vi "isProcessAllowedRun.vi"(8 "error in (no error)":errorcluster, 11 "SMO in":refnum<class "SMO.lvclass">) -> (0 "error out":errorcluster, 2 "Run Allowed":bool, 3 "SMO out":refnum<class "SMO.lvclass">)   [LabVIEW 2013, in "SMO.lvclass"]
uses:
  SMO.lvclass
  SMO.lvclass/SMO.ctl
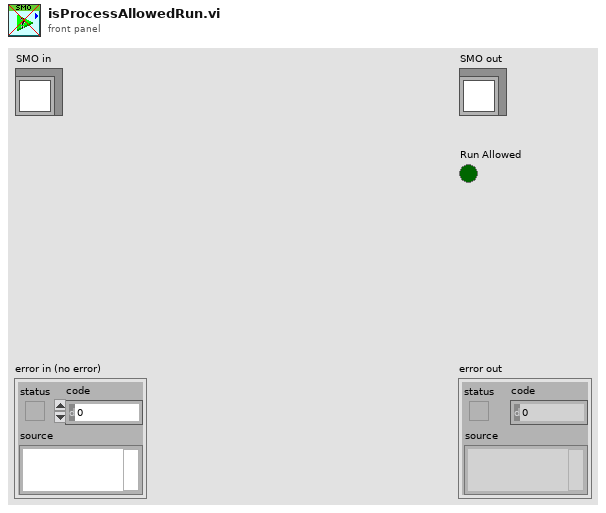
[diagram p1: front panel]
types:
  T1 = typedef "SMO.lvclass/PrivateData--Ref.ctl" = refnum<data-value>
  T2 = typedef "SMO.lvclass/PrivateData--Cluster.ctl" = cluster{"Parent Call":T3, "Registered Processes":T4[], "Sync Notifier":refnum<notifier>, "Process Error Notifier":refnum<notifier>, "Protected Events":T5, "Public Events":T6, "SMO State":T7, "[Dependencies]":T8[], "[Attributes]":refnum<class "Attribute.lvclass">[], "Launcher Close":refnum<notifier>}
  T3 = typedef "SMO.lvclass/Parent Call--Enum.ctl" = enum16{"Allows parent to run", "Does not request parent to run"}
  T4 = typedef "SMO.lvclass/RegisteredProcessData--Cluster.ctl" = cluster{"Name":string, "Static VI Ref":refnum<vi>, "Running":bool, "NotifierRef":u32}
  T5 = typedef "SMO.lvclass/Protected Events.ctl" = cluster{"StopProcesses":refnum<user-event>, "AbortProcesses":refnum<user-event>, "Config Changed":refnum<user-event>}
  T6 = typedef "SMO.lvclass/Public Events.ctl" = cluster{"Error":refnum<user-event>, "State":refnum<user-event>}
  T7 = typedef "SMO.lvclass/SMOState --Enum.ctl" = enum16{"unknown", "Created", "Started", "Stopped"}
  T8 = typedef "SMO.lvclass/SMO Dependency--Cluster.ctl" = cluster{"Dependency":refnum<class "SMO.lvclass">, "Level":string}
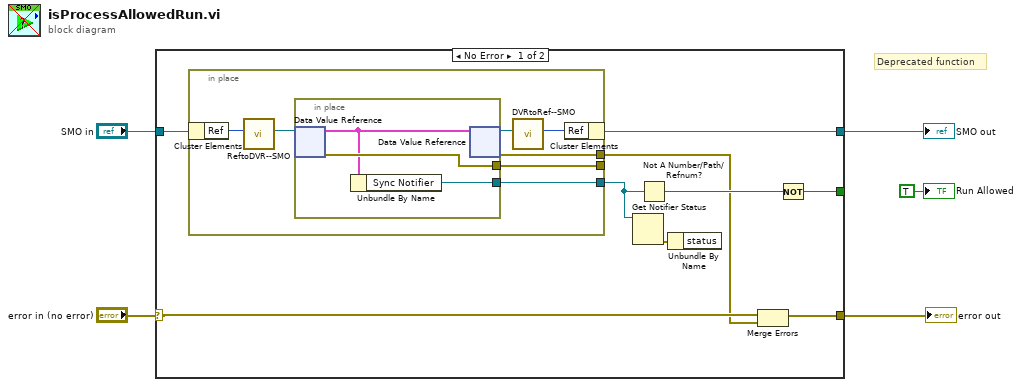
[diagram p0: block diagram]
diagram:
  # "Deprecated function"
  n1 = case shown="No Error" "error in (no error)" {
    selector: "error in (no error)" -> [w10 w26]
    tunnel: [w8 w26] -> w3
    tunnel: [w13 w25] -> w2
    tunnel: "SMO in" -> [w14 w25]
    tunnel: [w11 _] -> _
    frame No Error {
      n2 = in-place {
        in-place-border: [w21] -> w9
        in-place-border: [w20] -> _
        in-place-border: [w15] -> w7
        n3 = in-place-cluster #1(w14) -> ("Ref"=w19:u32)
        n4 = call "ReftoDVR--SMO.vi"("Ref"=w19) -> ("Ref"=w18:T1)  [unwired: 10 in]
        n5 = in-place {
          in-place-border: [w24] -> w20
          in-place-border: [w22] -> w15
          n6 = in-place-dvr #2(w18) -> (w23:T2, w24:errorcluster)
          n7 = Unbundle By Name(w23) -> ("Sync Notifier"=w22:refnum<notifier>)
          n8 = in-place-dvr #2(w23) -> (w17:T1, w21:errorcluster)
        }
        n9 = call "DVRtoRef--SMO.vi"("Ref"=w17) -> ("Ref"=w16:u32)  [unwired: 10 in]
        n10 = in-place-cluster #1("Ref"=w16) -> (w13:refnum<class "SMO.lvclass">)
      }
      n11 = Get Notifier Status(notifier=w7) -> (error out=w6:errorcluster)  [unwired: 1 in, 4 out]
      n12 = Not A Number/Path/Refnum?(number/path/refnum=w7) -> (NaN/Path/Refnum?=w12:bool)
      n13 = Unbundle By Name(w6) -> ()  [unwired: 1 out]
      n14 = Merge Errors(w10, w9) -> (w8:errorcluster)
      n15 = Not(x=w12) -> (.not. x?=w11:bool)
    }
    frame Error {
    }
  }
  "error out" <- w3
  "SMO out" <- w2
  "Run Allowed" <- TRUE ("Run Allowed")
